vi "SR430.get trig offset.vi"(0 "i ref in":refnum<vi>, 3 "ms timeout (10000)":i32=10000, 5 "error in (no error)":errorcluster) -> (14 "i ref out":refnum<vi>, 16 "triggerOffset [us]":i32, 17 "timed out":bool, 19 "error out":errorcluster)   [LabVIEW 2014, in "SR430.lvlib"]
doc: "Gets the Trigger Offset.\nThe value can go from 0 to 16384 per step of 16."
uses:
  SR430.lvlib
  CS_Core/CSSystem/CoreDefs/CoreDefs.error_type.ctl
  instr.lib/SR430/SR430Driver.lvlib
  CS_Core/CSSystem/CoreLib/CoreLib.lvlib
  CSlibraries/UtilityLib/UtilityLib.lvlib
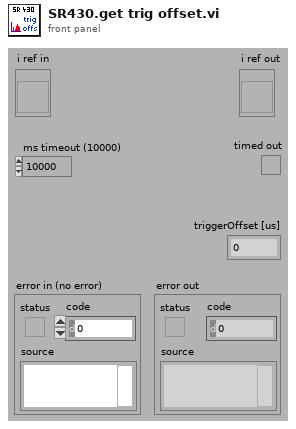
[diagram p1: front panel]
types:
  T1 = typedef "CoreDefs.error_type.ctl" = enum16{"no error", "can't load process", "can't unload process", "process does not exist", "can't install process", "can't remove process", "unknown function", "time out", "can't execute function", "duplicate queue name", "super not found", "caller queue invalid", "can't ping process", "unknown error", "VISA Error", "VISA timeout", "GPIB timeout", "GPIB error", "communication error", "data type mismatch", "can't read data from OPC server", "can't write data to OPC server", "OET error", "function not implemented", "process already exists", "invalid Shared Variable name", "error writing Shared Variable", "error reading Shared Variable", "invalid client name", "corrupt database", "unknown class", "call not authorized", "parameter out of range", "OET timeout: can't get data to modify", "invalid queue name", "requested operation incompatible with current state", "event undefined", "event disabled", "state undefined", "caller is not a friend", "EventBuilder: bad eventID", "EventBuilder: no DAQ devices", "a thread must not stop itself", "UNUSED ELEMENT4", "DiscArchiver: eventData incomplete", "DiscArchiver: eventData does not belong to run", "DiscArchiver: can't open file", "DiscArchiver: can't write to file", "DiscArchiver: available disc space low", "can't acquire semaphore", "error reading data from database", "notifier object is not existing", "can't register process", "can't unregister process", "illegal event type", "object disabled", "object already exists", "can't change state", "Instrument not found", "no connection to remote node", "invalid reference", "N/A", "UNUSED ELEMENT 1", "element not found", "illegal TCP/IP connection detected", "object does not exist", "invalid access ID", "unknown CS system", "invalid privilige", "unsupported data type", "unsupported server type", "IO server already exists", "Shared Variable already exists"}
  T2 = typedef "SR430Driver.lvlib/SR430_VISA Control.ctl" = cluster{"VISA resource name":refnum<visa-resource-name>}
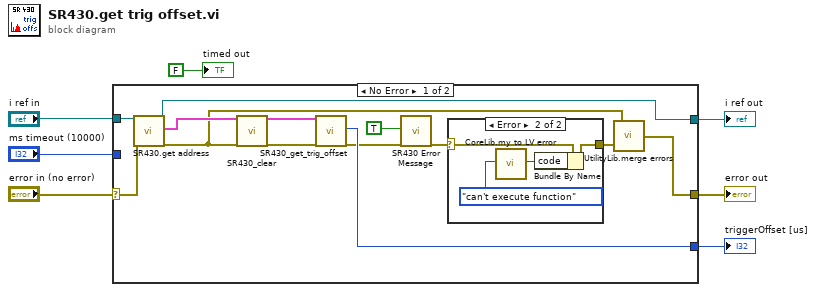
[diagram p0: block diagram]
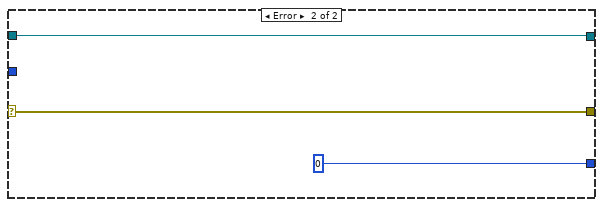
[diagram p3: hidden frame]
diagram:
  n1 = case shown="No Error" "error in (no error)" {
    selector: "error in (no error)" -> [w8 w26]
    tunnel: "i ref in" -> [w20 w27]
    tunnel: [w17 w26] -> w6
    tunnel: [w16 w27] -> w5
    tunnel: [w15 0] -> w4
    tunnel: "ms timeout (10000)" -> [_ _]
    frame No Error {
      n2 = call "SR430.get address.vi"("i ref in"=w20, "error in (no error)"=w8) -> ("i ref out"=w16:refnum<vi>, "address"=w19:T2, "error out"=w18:errorcluster)  [unwired: 15 in]
      n3 = call "SR430_clear.vi"("address"=w19, "error in (no error)"=w18) -> ("address out"=w9:T2, "error out"=w10:errorcluster)  [unwired: 16 in]
      n4 = call "SR430_get_trig_offset.vi"("address"=w9, "error in (no error)"=w10) -> ("triggerOffset"=w15:i32, "error out"=w11:errorcluster)  [unwired: 15 in, 1 out]
      n5 = call "SR430 Error Message.vi"("addMessageToSource"=TRUE ("add message to source"), "error in (no error)"=w11) -> ("error out"=w14:errorcluster)  [unwired: 14 in, 3 out]
      n6 = case shown="Error" w14 {
        selector: w14 -> [w21 w25]
        tunnel: [w21 w22] -> w12
        frame No Error {
        }
        frame Error {
          n7 = call "CoreLib.my to LV error.vi"("ErrorTypes"=CoreDefs.error_type."can't execute function") -> ("LV error code"=w24:i32)  [unwired: 17 in, 1 out]
          n8 = Bundle By Name(cluster=w25, "code"=w24) -> (w22:errorcluster)
        }
      }
      n9 = call "UtilityLib.merge errors.vi"("error2 (no error)"=w12, "error1 (no error)"=w18) -> ("error out"=w17:errorcluster)
    }
    frame Error {
    }
  }
  "error out" <- w6
  "i ref out" <- w5
  "triggerOffset [us]" <- w4
  "timed out" <- FALSE ("timed out")
